vi "pressure-tdms-file-explorer.vi"() -> ()   [LabVIEW 2016]
panel:
  in  "stop":bool
  out "Waveform Graph":dynamicdata(graph)
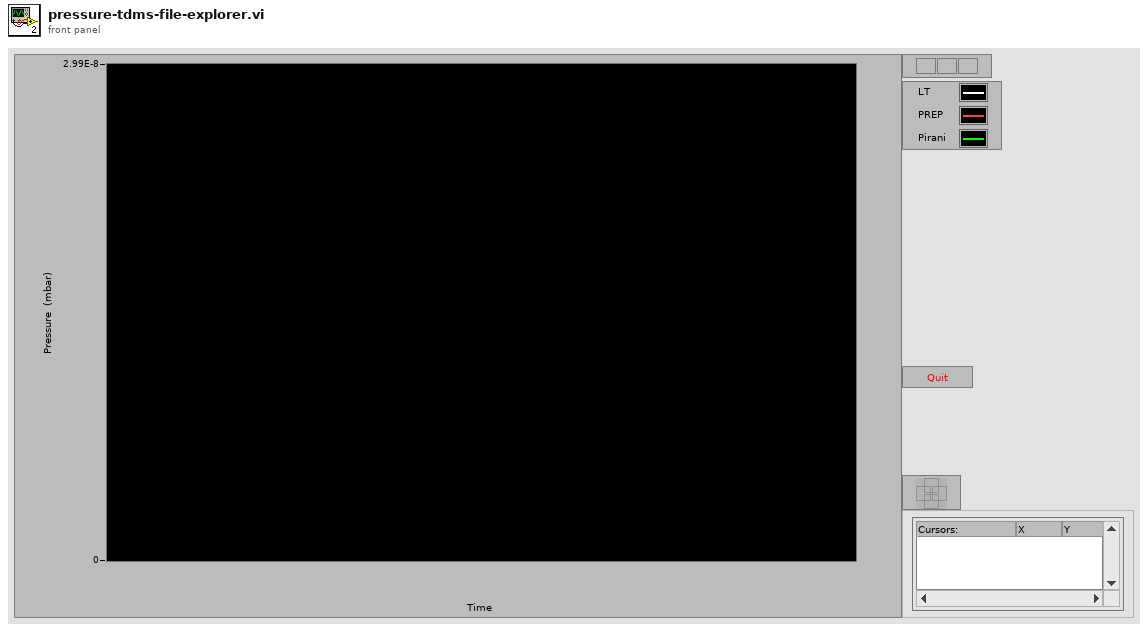
[diagram p1: front panel]
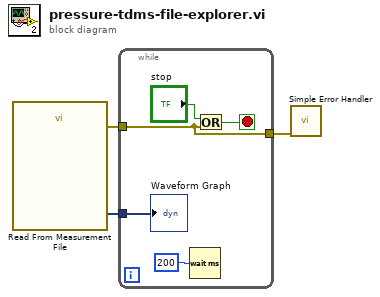
[diagram p0: block diagram]
diagram:
  n1 = call "Read From Measurement File"() -> ("error out"=w2:errorcluster, "Signals"=w3:dynamicdata)  [unwired: 6 in, 4 out]
  n2 = while {
    tunnel: w3 -> [w6]
    tunnel: w2 -> [w4]
    tunnel: [w4] -> w1
    stop <- w5 stop-if-true
    n3 = Wait (ms)(milliseconds to wait=u32 200) -> ()  [unwired: 1 out]
    n4 = Or(x="stop", y=w4) -> (x .or. y?=w5:bool)
    "Waveform Graph" <- w6
  }
  n5 = call <vilib>:"Simple Error Handler.vi"("error in (no error)"=w1) -> ()  [unwired: 4 in, 5 out]
